vi "Main.vi"() -> ()   [LabVIEW 2019]
uses:
  Lib/TypeDef/File Type.ctl
  Lib/TypeDef/App State.ctl
  Lib/TypeDef/App Data.ctl
panel:
  in  "FilterType":enum32{"Butterworth"}(tab)
  out "Samples Number":dbl
  in  "Sampling Freq.":dbl format="%#_g Hz"
  in  "FileType":T1
  in  "Group Name":string(combo)
  in  "Channel Name":string(combo)
  in  "Data Path":path
  in  "ReadFile":bool
  in  "Panel":T2(tab)
  out "Filter Impulse Response":dbl[](graph)
  out "Impulse Signal":dbl[](graph)
  out "RAW Signal":dbl[](graph)
  in  "Stop":bool
  # "Filter Parameters Fitting App"
  # "File Parameters"
  # "Filter Parameters"
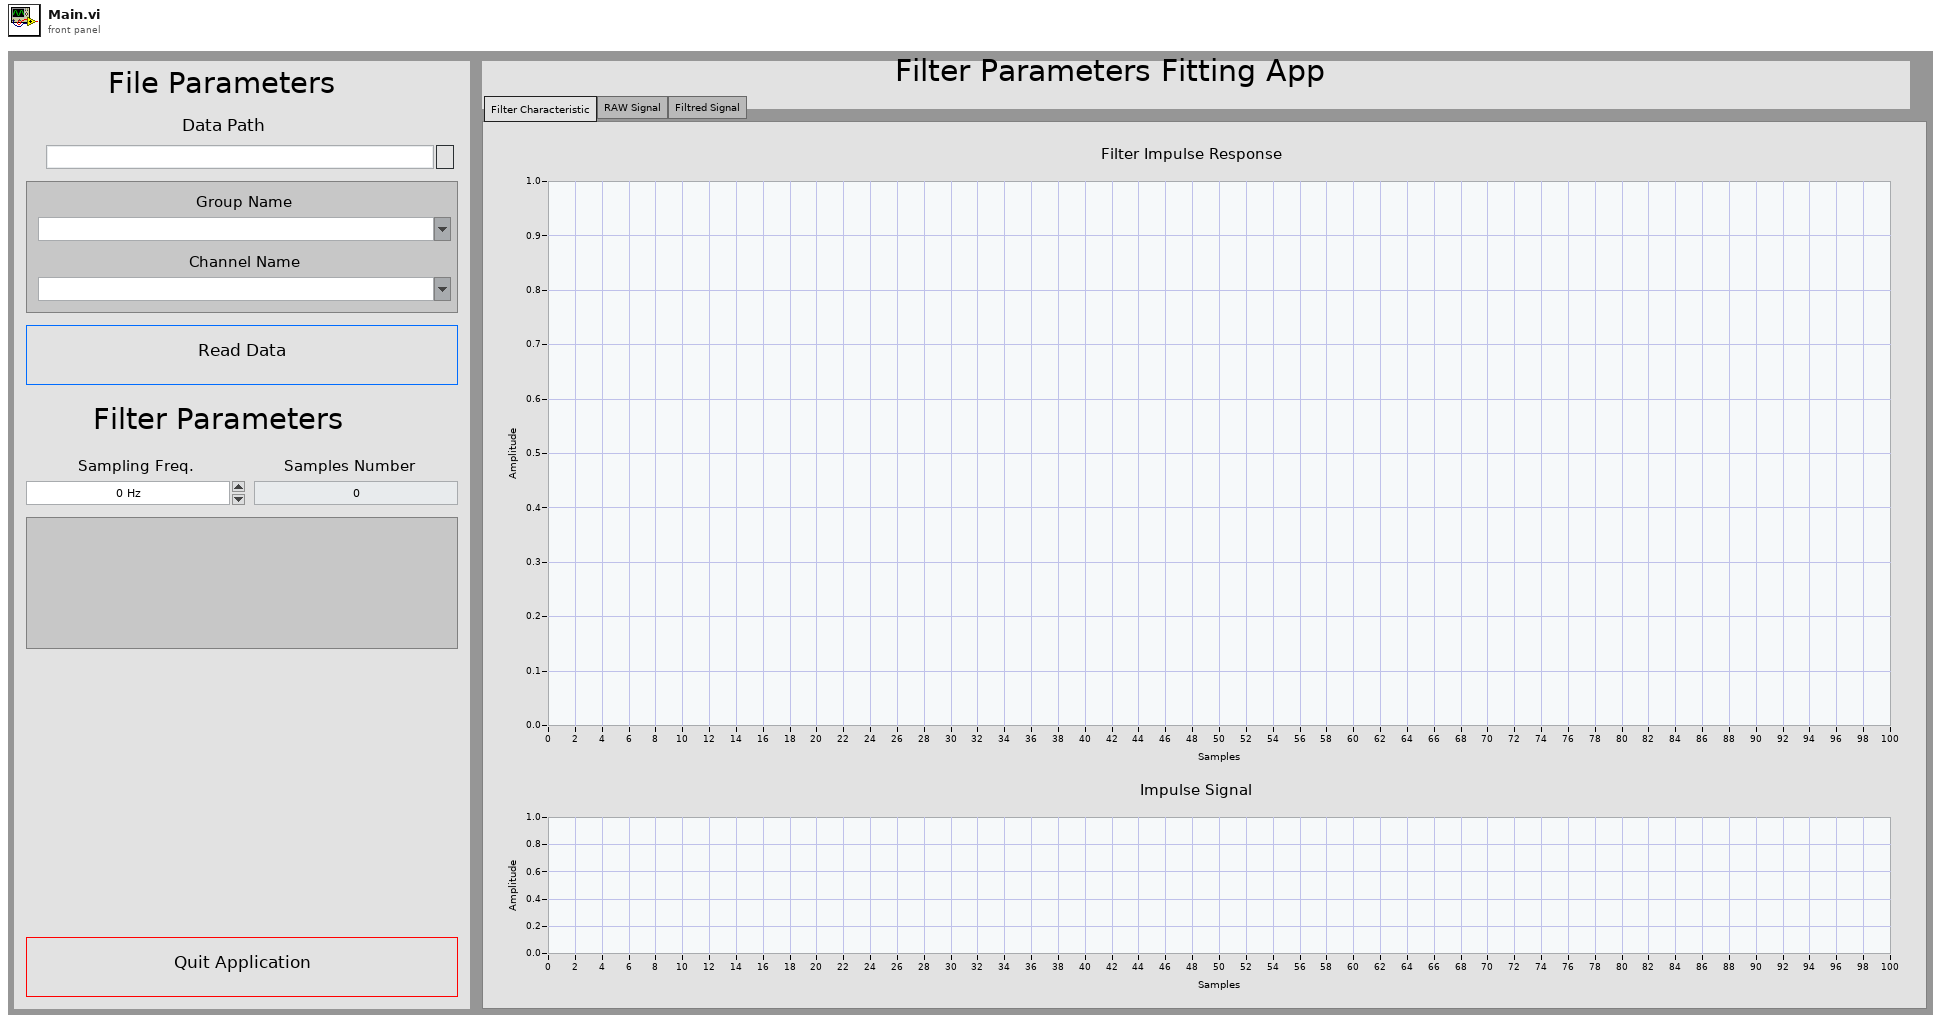
[diagram p1: front panel]
types:
  T1 = typedef "File Type.ctl" = enum32{"TDMS", "CSV"}
  T2 = enum32{"Filter Characteristic", "RAW Signal", "Filtred Signal"}
  T3 = typedef "App Data.ctl" = cluster{"UI":cluster{"Panel":refnum<vi>, "Data Path":refnum<vi>, "FileType":refnum<vi>, "ReadFile":refnum<vi>, "FilterType":refnum<vi>, "Sampling Freq.":refnum<vi>, "Samples Number":refnum<vi>, "TDMS":cluster{"Group Name":refnum<vi>, "Channel Name":refnum<vi>}}, "File":cluster{"TDMS REF":refnum<k34>}}
  T4 = typedef "App State.ctl" = enum16{"Init", "LoadFile", "LoadDataFromFile", "RunFilter", "GenerateRaport", "Exit"}
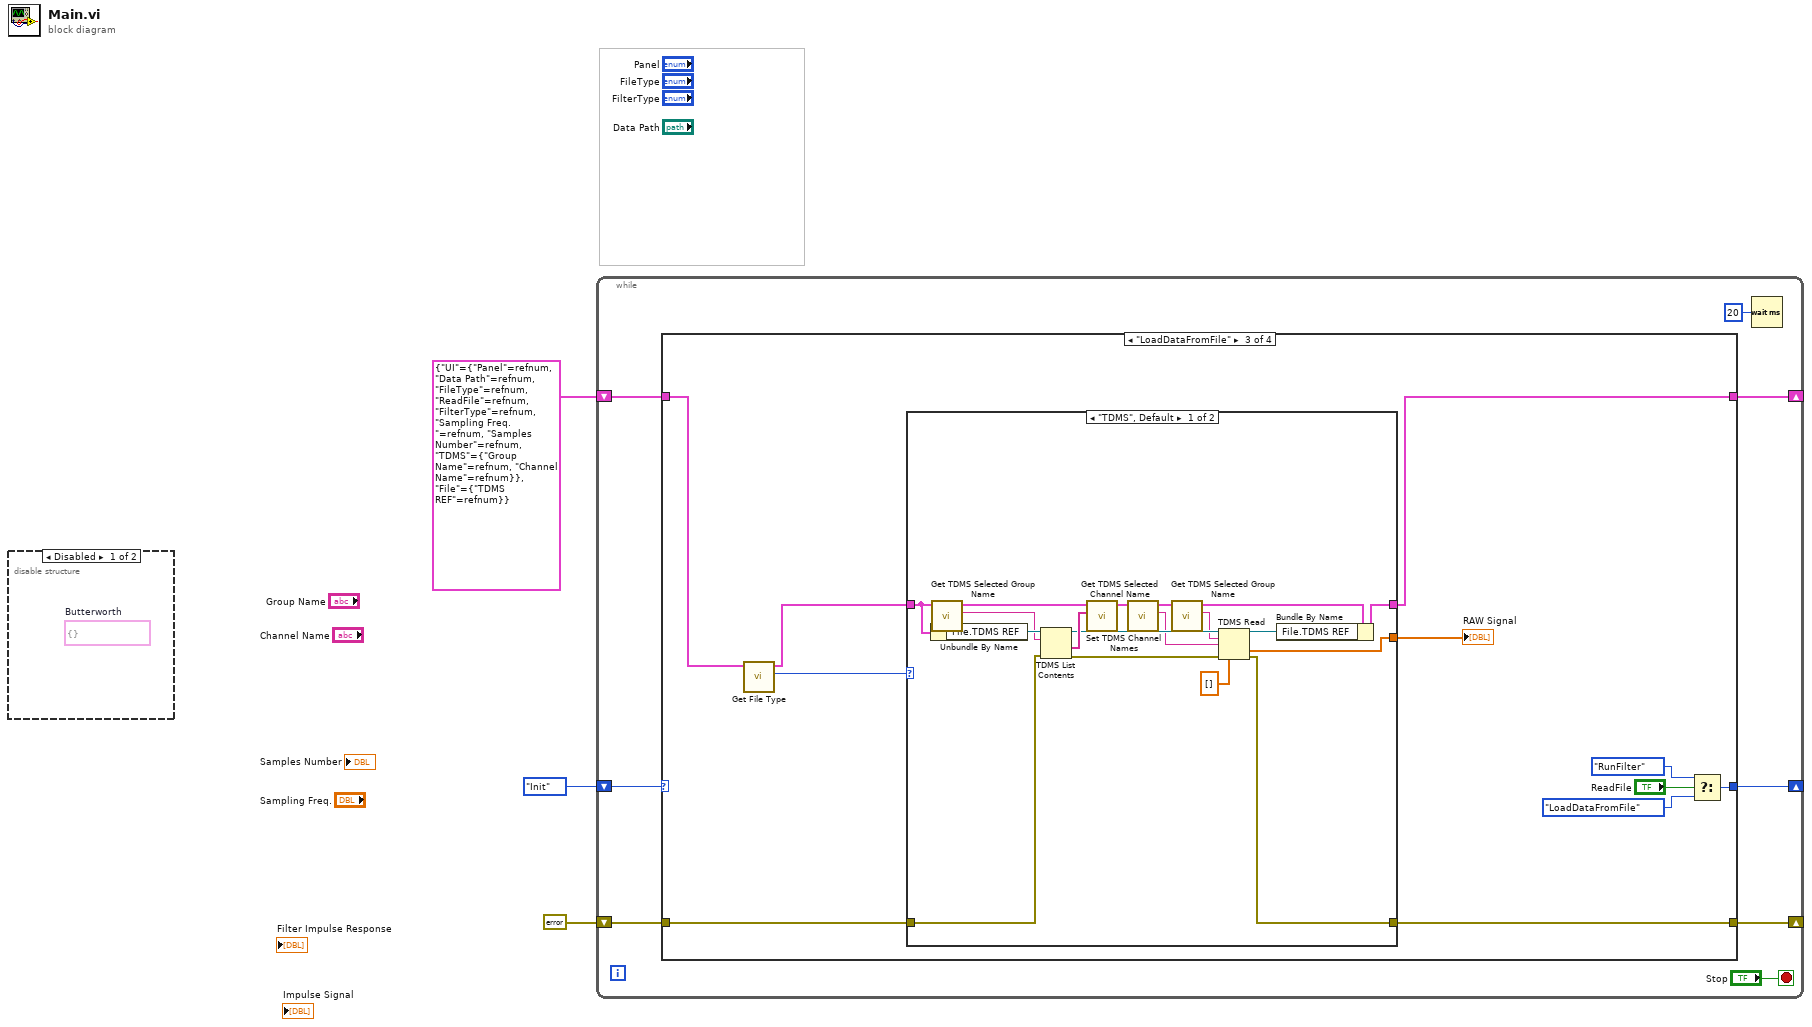
[diagram p0: block diagram]
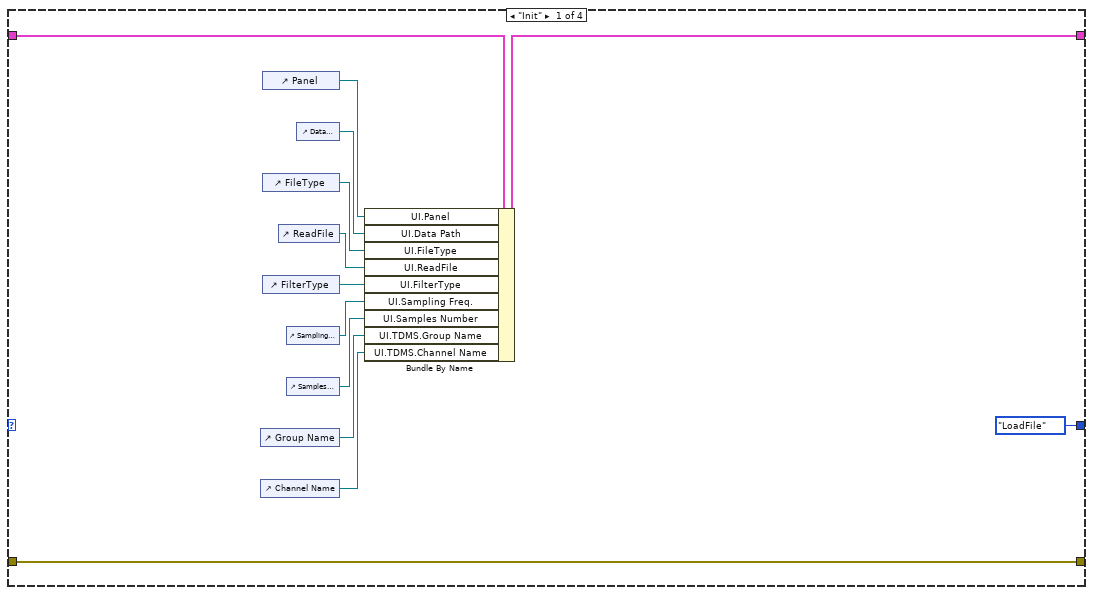
[diagram p3: hidden frame]
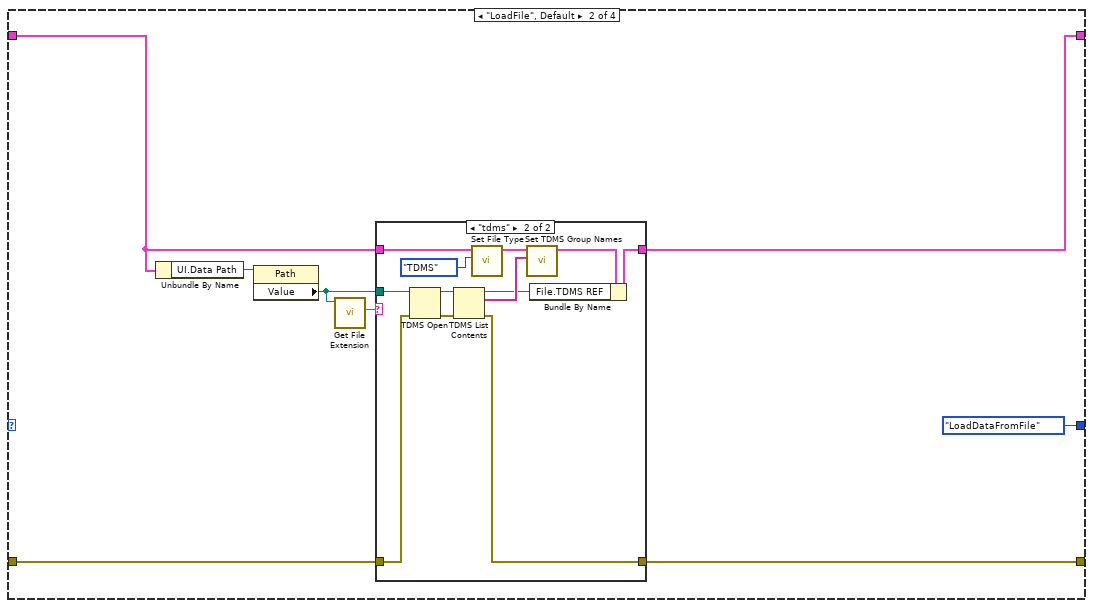
[diagram p4: hidden frame]
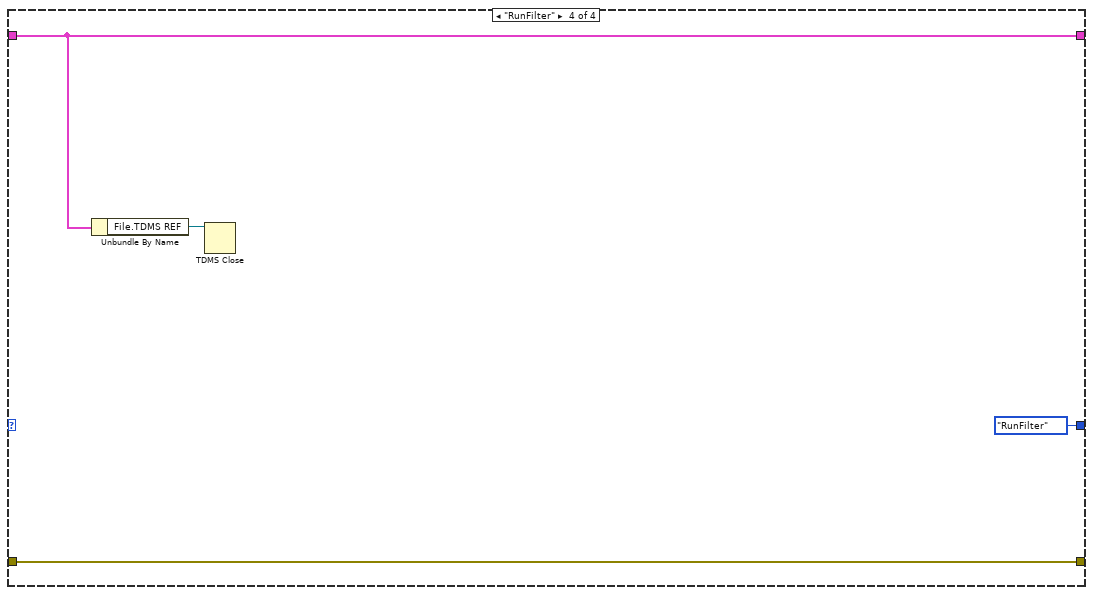
[diagram p7: hidden frame]
diagram:
  n1 = disable-structure shown="Disabled" {
    frame Disabled {
      (unwired) cluster{} {}  # Butterworth
    }
    frame Enabled {
    }
  }
  n2 = while {
    shift-right: [w8] -> _
    shift-left: T3 {"UI"={"Panel"=refnum, "Data Path"=refnum, "FileType"=refnum, "ReadFile"=refnum, "FilterType"=refnum, "Sampling Freq."=refnum, "Samples Number"=refnum, "TDMS"={"Group Name"=refnum, "Channel Name"=refnum}}, "File"={"TDMS REF"=refnum}} -> [w9]
    shift-right: [w6] -> _
    shift-left: App_State."Init" -> [w11]
    shift-right: [w4] -> _
    shift-left: errorcluster {"status"=FALSE, "code"=0, "source"=""} ("error constant") -> [w5]
    stop <- "Stop" stop-if-true
    n3 = case shown="\"LoadDataFromFile\"" w11 {
      tunnel: w9 -> [w24 w26 w57 w79]
      tunnel: [w23 w27 w47 w79] -> w8
      tunnel: [App_State."LoadFile" App_State."LoadDataFromFile" w53 App_State."RunFilter"] -> w6
      tunnel: w5 -> [w12 w29 w55 w81]
      tunnel: [w12 w28 w56 w81] -> w4
      frame "Init" {
        n4 = control-ref of="Group Name"() -> (w16:refnum<vi>)
        n5 = control-ref of="Channel Name"() -> (w15:refnum<vi>)
        n6 = control-ref of="Panel"() -> (w22:refnum<vi>)
        n7 = control-ref of="FileType"() -> (w13:refnum<vi>)
        n8 = control-ref of="FilterType"() -> (w19:refnum<vi>)
        n9 = control-ref of="ReadFile"() -> (w20:refnum<vi>)
        n10 = control-ref of="Sampling Freq."() -> (w18:refnum<vi>)
        n11 = control-ref of="Samples Number"() -> (w17:refnum<vi>)
        n12 = control-ref of="Data Path"() -> (w21:refnum<vi>)
        n13 = Bundle By Name(cluster=w24, "UI.Panel"=w22, "UI.Data Path"=w21, "UI.FileType"=w13, "UI.ReadFile"=w20, "UI.FilterType"=w19, "UI.Sampling Freq."=w18, "UI.Samples Number"=w17, "UI.TDMS.Group Name"=w16, "UI.TDMS.Channel Name"=w15) -> (w23:T3)
      }
      frame "LoadFile", Default {
        n14 = Unbundle By Name(w26) -> ("UI.Data Path"=w32:refnum<vi>)
        n15 = property class="Path"(reference=w32) -> ("Value"=w30:path)  [unwired: 1 in, 2 out]
        n16 = call <vilib>:"Get File Extension.vi"("file"=w30) -> ("lowercase file extension"=w31:string)  [unwired: 6 in, 4 out]
        n17 = case shown="\"tdms\"" w31 {
          tunnel: w30 -> [_ w46]
          tunnel: w29 -> [w34 w45]
          tunnel: [w34 w35] -> w28
          tunnel: [w33 w38] -> w27
          tunnel: w26 -> [w33 w44]
          frame Default {
          }
          frame "tdms" {
            n18 = TDMS Open(8:w45, 11:w46) -> (0:w41:errorcluster, 3:w42:refnum<k34>)  [unwired: 5 in]
            n19 = TDMS List Contents(4:w41, 7:w42) -> (0:w35:errorcluster, 2:w39:string[], 3:w36:refnum<k34>)  [unwired: 1 in, 1 out]
            n20 = call "Set File Type.vi"("Value"=File_Type."TDMS" ("FileType"), "App Data In"=w44) -> ("App Data Out"=w40:T3)  [unwired: 9 in]
            n21 = call "Set TDMS Group Names.vi"("Group Names"=w39, "App Data In"=w40) -> ("App Data Out"=w37:T3)  [unwired: 9 in]
            n22 = Bundle By Name(cluster=w37, "File.TDMS REF"=w36) -> (w38:T3)
          }
        }
      }
      frame "LoadDataFromFile" {
        n23 = call "Get File Type.vi"("App Data In"=w57) -> ("FileType"=w54:T1, "App Data Out"=w49:T3)  [unwired: 9 in]
        n24 = case shown="\"TDMS\", Default" w54 {
          tunnel: [w62 w77] -> w56
          tunnel: w55 -> [w63 w77]
          tunnel: w49 -> [w75 w76]
          tunnel: [w61 _] -> w48
          tunnel: [w59 w76] -> w47
          frame "TDMS", Default {
            n25 = Unbundle By Name(w75) -> ("File.TDMS REF"=w74:refnum<k34>)
            n26 = call "Get TDMS Selected Group Name.vi"("App Data In"=w75) -> ("Selected Group Name"=w73:string, "App Data Out"=w72:T3)  [unwired: 9 in]
            n27 = TDMS List Contents(4:w63, 6:w73, 7:w74) -> (0:w64:errorcluster, 1:w71:string[], 3:w69:refnum<k34>)  [unwired: 1 out]
            n28 = call "Set TDMS Channel Names.vi"("Channel Names"=w71, "App Data In"=w72) -> ("App Data Out"=w70:T3)  [unwired: 9 in]
            n29 = call "Get TDMS Selected Channel Name.vi"("App Data In"=w70) -> ("Selected Channel Name"=w67:string, "App Data Out"=w68:T3)  [unwired: 9 in]
            n30 = call "Get TDMS Selected Group Name.vi"("App Data In"=w68) -> ("Selected Group Name"=w66:string, "App Data Out"=w60:T3)  [unwired: 9 in]
            n31 = TDMS Read(0:w69, 5:w66, 7:w67, 11:w64, 12:dbl[] []) -> (4:w58:refnum<k34>, 10:w61:dbl[], 15:w62:errorcluster)  [unwired: 3 in, 3 out]
            n32 = Bundle By Name(cluster=w60, "File.TDMS REF"=w58) -> (w59:T3)
          }
          frame "CSV" {
          }
        }
        "RAW Signal" <- w48
        n33 = Select(t=App_State."RunFilter", s="ReadFile", f=App_State."LoadDataFromFile") -> (s? t:f=w53:T4)
      }
      frame "RunFilter" {
        n34 = Unbundle By Name(w79) -> ("File.TDMS REF"=w78:refnum<k34>)
        n35 = TDMS Close(11:w78) -> ()  [unwired: 1 in, 2 out]
      }
    }
    n36 = Wait (ms)(milliseconds to wait=u32 20) -> ()  [unwired: 1 out]
  }
